vi "Create ARGB Test Image.vi"(8 "error in (no error)":errorcluster, 11 "Preallocated Image Size":T1) -> (0 "error out":errorcluster, 2 "24-bit pixmap":u32[][](array[numeric]), 3 "Data Value Reference out":refnum<data-value>)   [LabVIEW 2020, in "g_ar_toolkit.test.lvlib" / "Image.lvclass"]
uses:
  g_ar_toolkit.test/Image/Image.lvclass
  g_ar_toolkit.test/Image/Image.lvclass/Image.ctl
  g_ar_toolkit.image.lvlib
  CreateEmptyImageARGB.vi
  Image Size (Fixed).ctl
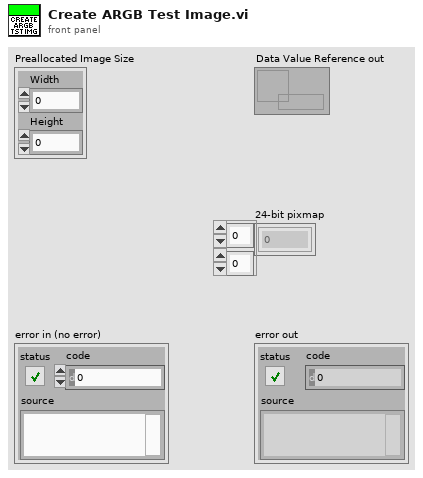
[diagram p1: front panel]
types:
  T1 = typedef "g_ar_toolkit.image.lvlib/Image Size (Fixed).ctl" = cluster{"Width":u16, "Height":u16}
  T2 = typedef "imagedata.ctl" = cluster{"image type":i32, "image depth":i32, "image":u8[], "mask":u8[], "colors":u32[], "Rectangle":cluster{"left":i16, "top":i16, "right":i16, "bottom":i16}}
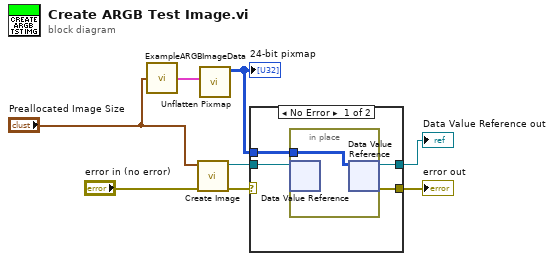
[diagram p0: block diagram]
diagram:
  n1 = call "ExampleARGBImageData.vi"("Image Size"="Preallocated Image Size") -> ("RGB Image Data"=w7:T2)
  n2 = call-poly "Create Image.vi"("error in (no error)"="error in (no error)", "Preallocated Image Size (Default: 0,0)"="Preallocated Image Size") -> ("error out"=w4:errorcluster, "New ARGB Image"=w3:refnum<data-value>)  [unwired: 8 in]
  n3 = call <vilib>:"Unflatten Pixmap.vi"("image data"=w7) -> ("24-bit pixmap"=w6:u32[][])  [unwired: 4 in, 6 out]
  "24-bit pixmap" <- w6
  n4 = case shown="No Error" w4 {
    selector: w4 -> [_ w14]
    tunnel: w3 -> [w12 w15]
    tunnel: [w11 w15] -> w8
    tunnel: [w10 w14] -> w5
    tunnel: w6 -> [w9 _]
    frame No Error {
      n5 = in-place {
        in-place-border: w9 -> [w13]
        n6 = in-place-dvr #1(w12) -> ()  [unwired: 2 out]
        n7 = in-place-dvr #1(w13) -> (w11:refnum<data-value>, w10:errorcluster)
      }
    }
    frame Error {
    }
  }
  "Data Value Reference out" <- w8
  "error out" <- w5
